vi "SelectPatternDialog.vi"(0 "GraphIn":refnum<class "Graph.lvclass">, 1 "SelectedNodes":refnum<class "AbstractNode.lvclass">[](array[class]), 5 "error in":errorcluster) -> (14 "GraphOut":refnum<class "Graph.lvclass">, 15 "Cancelled":bool, 16 "NodesOut":T3[](array[typedef]), 17 "LinksOut":T1[](array[typedef]), 18 "NodeIndexies":i32[](array[numeric]), 19 "error out":errorcluster)   [LabVIEW 2012]
uses:
  <resource>/Framework/Providers/Open_GDS/UML/Graph_class/Graph.lvclass
  <resource>/Framework/Providers/Open_GDS/UML/AbstractNode_class/AbstractNode.lvclass
  <resource>/Framework/Providers/Open_GDS/UML/DesignPattern/SubVIs/DesignPatterns_Node.ctl
  <resource>/Framework/Providers/Open_GDS/UML/DesignPattern/SubVIs/DesignPatterns_NodeType.ctl
  <resource>/Framework/Providers/Open_GDS/UML/DesignPattern/SubVIs/DesignPatterns_Link.ctl
  <resource>/Framework/Providers/Open_GDS/UML/DesignPattern/SubVIs/DesignPatterns_LinkType.ctl
  <resource>/Framework/Providers/Open_GDS/UML/Graphics_class/Graphics.lvclass
  <resource>/Framework/Providers/Open_GDS/UML/Grid_class/Grid.lvclass
  <resource>/Framework/Providers/Open_GDS/UML/ClassDiagramGraph_class/ClassDiagramGraph.lvclass
  <resource>/Framework/Providers/Open_GDS/UML/DesignPattern/SubVIs/DesignPatterns_Pattern.ctl
  <resource>/Framework/Providers/Open_GDS/UML/ClassNode_class/ClassNode.lvclass
  <resource>/Framework/Providers/Open_GDS/UML/Graphics_class/LvFontType.ctl
  <resource>/Framework/Providers/Open_GDS/UML/Graphics_class/FontType.ctl
  <resource>/Framework/Providers/Open_GDS/UML/DesignPattern/SubVIs/DesignPatterns_ClassNodeData.ctl
  <resource>/Framework/Providers/Open_GDS/UML/DesignPattern/SubVIs/DesignPatterns_Attribute.ctl
  <resource>/Framework/Providers/Open_GDS/UML/DesignPattern/SubVIs/DesignPatterns_Method.ctl
  <vilib>/Platform/browser.llb/Open URL in Default Browser (string).vi
panel:
  in  "OpenPatternFile":bool
  in  "Refresh":bool
  in  "Ring 10":u16(ring) items=["<Select>", "Handler", "ConcreteHandler1", "ConcreteHandler2", "Client"]
  in  "Ring 9":u16(ring) items=["<Select>", "Handler", "ConcreteHandler1", "ConcreteHandler2", "Client"]
  in  "Ring 8":u16(ring) items=["<Select>", "Handler", "ConcreteHandler1", "ConcreteHandler2", "Client"]
  in  "Ring 7":u16(ring) items=["<Select>", "Handler", "ConcreteHandler1", "ConcreteHandler2", "Client"]
  in  "Help":bool
  in  "Cancel":bool
  in  "OK":bool
  out "Nodes":cluster{"Name":string, "Desc":string}[](array[cluster])
  out "Pattern description":string
  out "NewVal":string
  in  "Design Patterns":string(tree)
  in  "InterfaceNames":string[](array[string])
  in  "PackageNames":string[](array[string])
  out "ClassNames":string[](array[string])
  in  "Ring 6":u16(ring) items=["<Select>", "Handler", "ConcreteHandler1", "ConcreteHandler2", "Client"]
  in  "Ring 5":u16(ring) items=["<Select>", "Handler", "ConcreteHandler1", "ConcreteHandler2", "Client"]
  in  "Ring 4":u16(ring) items=["<Select>", "Handler", "ConcreteHandler1", "ConcreteHandler2", "Client"]
  in  "Ring 3":u16(ring) items=["<Select>", "Handler", "ConcreteHandler1", "ConcreteHandler2", "Client"]
  in  "Ring 2":u16(ring) items=["<Select>", "Handler", "ConcreteHandler1", "ConcreteHandler2", "Client"]
  in  "Ring 1":u16(ring) items=["<Select>", "Handler", "ConcreteHandler1", "ConcreteHandler2", "Client"]
  out "Picture":picture
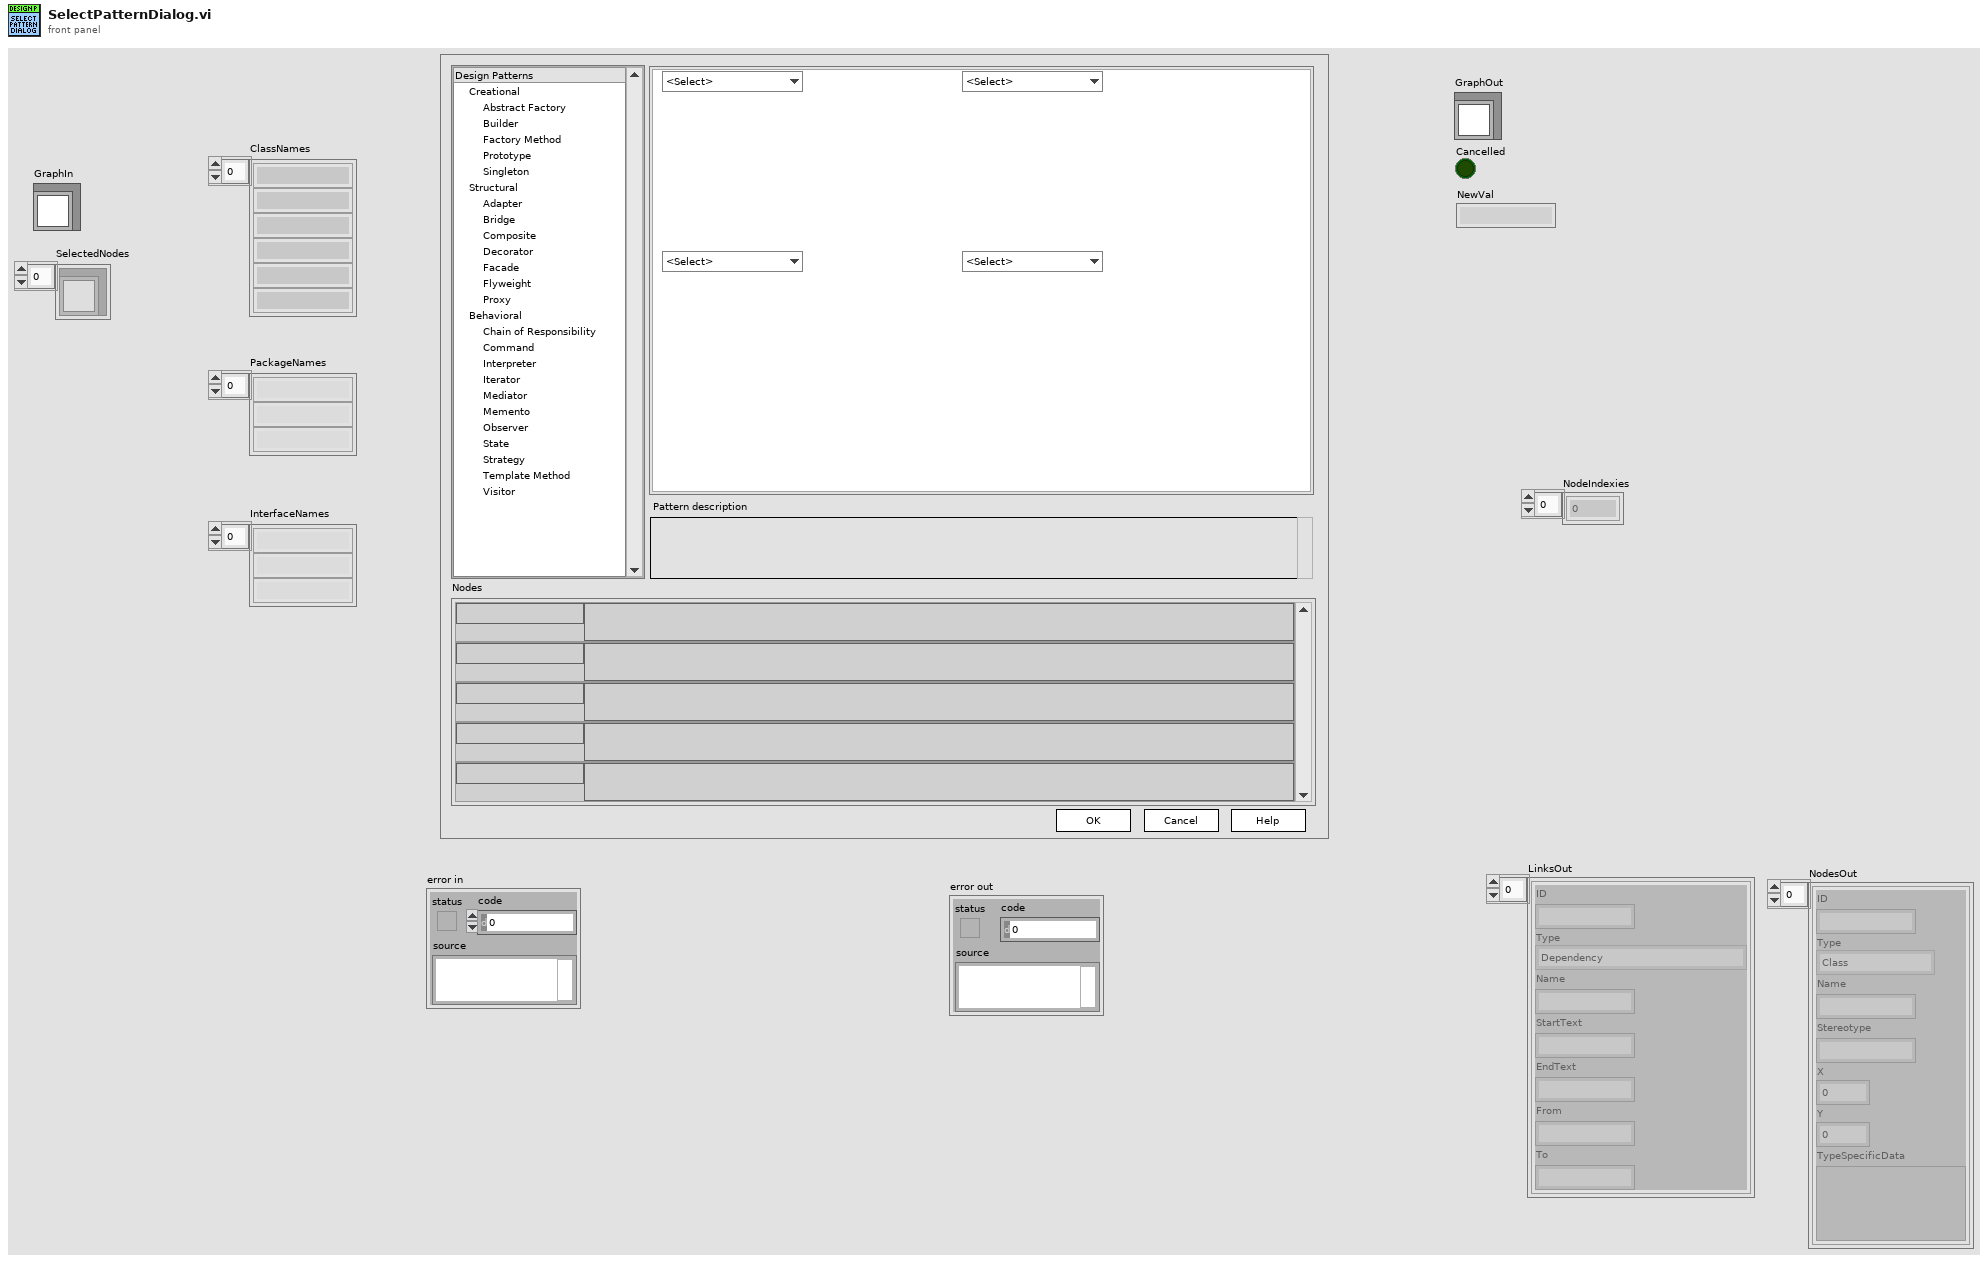
[diagram p1: front panel]
types:
  T1 = typedef "DesignPatterns_Link.ctl" = cluster{"ID":string, "Type":T2, "Name":string, "StartText":string, "EndText":string, "From":string, "To":string}
  T2 = typedef "DesignPatterns_LinkType.ctl" = enum16{"Dependency", "Inheritance", "Interface", "Association", "Aggregation", "CompositeAggregation"}
  T3 = typedef "DesignPatterns_Node.ctl" = cluster{"ID":string, "Type":T4, "Name":string, "Stereotype":string, "X":i32, "Y":i32, "TypeSpecificData":variant}
  T4 = typedef "DesignPatterns_NodeType.ctl" = enum16{"Class", "Interface", "Note", "Package"}
  T5 = typedef "DesignPatterns_Pattern.ctl" = cluster{"Version":string, "ID":string, "Name":string, "Category":string, "Help":string, "Desc":string}
  T6 = cluster{"Cancelled":bool, "Event":refnum<event-registration>, "CtrlRefs":refnum<vi>[], "PIDs":string[], "Graphics":refnum<class "Graphics.lvclass">, "Grid":refnum<class "Grid.lvclass">, "Diagram":refnum<class "ClassDiagramGraph.lvclass">, "ClassNodes":T3[], "ClassSelected":bool[], "NodeIndexies":i32[], "Patterns":cluster{"PatternFile":path, "Pattern":T5, "Nodes":T3[], "Links":T1[], "stripped path":path, "HelpExist":bool}[]}
  T7 = typedef "Graphics.lvclass/FontType.ctl" = cluster{"Font Name:":string, "Size":i16, "Strikeout?":bool, "Italic?":bool, "Underline?":bool, "Outline?":bool, "Shadow?":bool, "Bold?":bool}
  T8 = typedef "Graphics.lvclass/LvFontType.ctl" = enum16{"User-specified Font", "Application Font", "System Font", "Dialog Font"}
  T9 = cluster{path, "Pattern":T5, "Nodes":T3[], "Links":T1[], "stripped path":path, "file or folder exists?":bool}[]
  T10 = typedef "DesignPatterns_ClassNodeData.ctl" = cluster{"Description":string, "Attributes":T11[], "Methods":T12[]}
  T11 = typedef "DesignPatterns_Attribute.ctl" = cluster{"ID":string, "Name":string}
  T12 = typedef "DesignPatterns_Method.ctl" = cluster{"ID":string, "Name":string}
  T13 = typedef "Rectangle Rectangle2D.ctl" = cluster{"x":dbl, "y":dbl, "width":dbl, "height":dbl}
  T14 = cluster{path, "Pattern":T5, "Nodes":T3[], "Links":T1[], "stripped path":path, "file or folder exists?":bool}
  T15 = cluster{"PatternFile":path, "Pattern":T5, "Nodes":T3[], "Links":T1[], "stripped path":path, "HelpExist":bool}[]
  T16 = cluster{"PatternFile":path, "Pattern":T5, "Nodes":T3[], "Links":T1[], "stripped path":path, "HelpExist":bool}
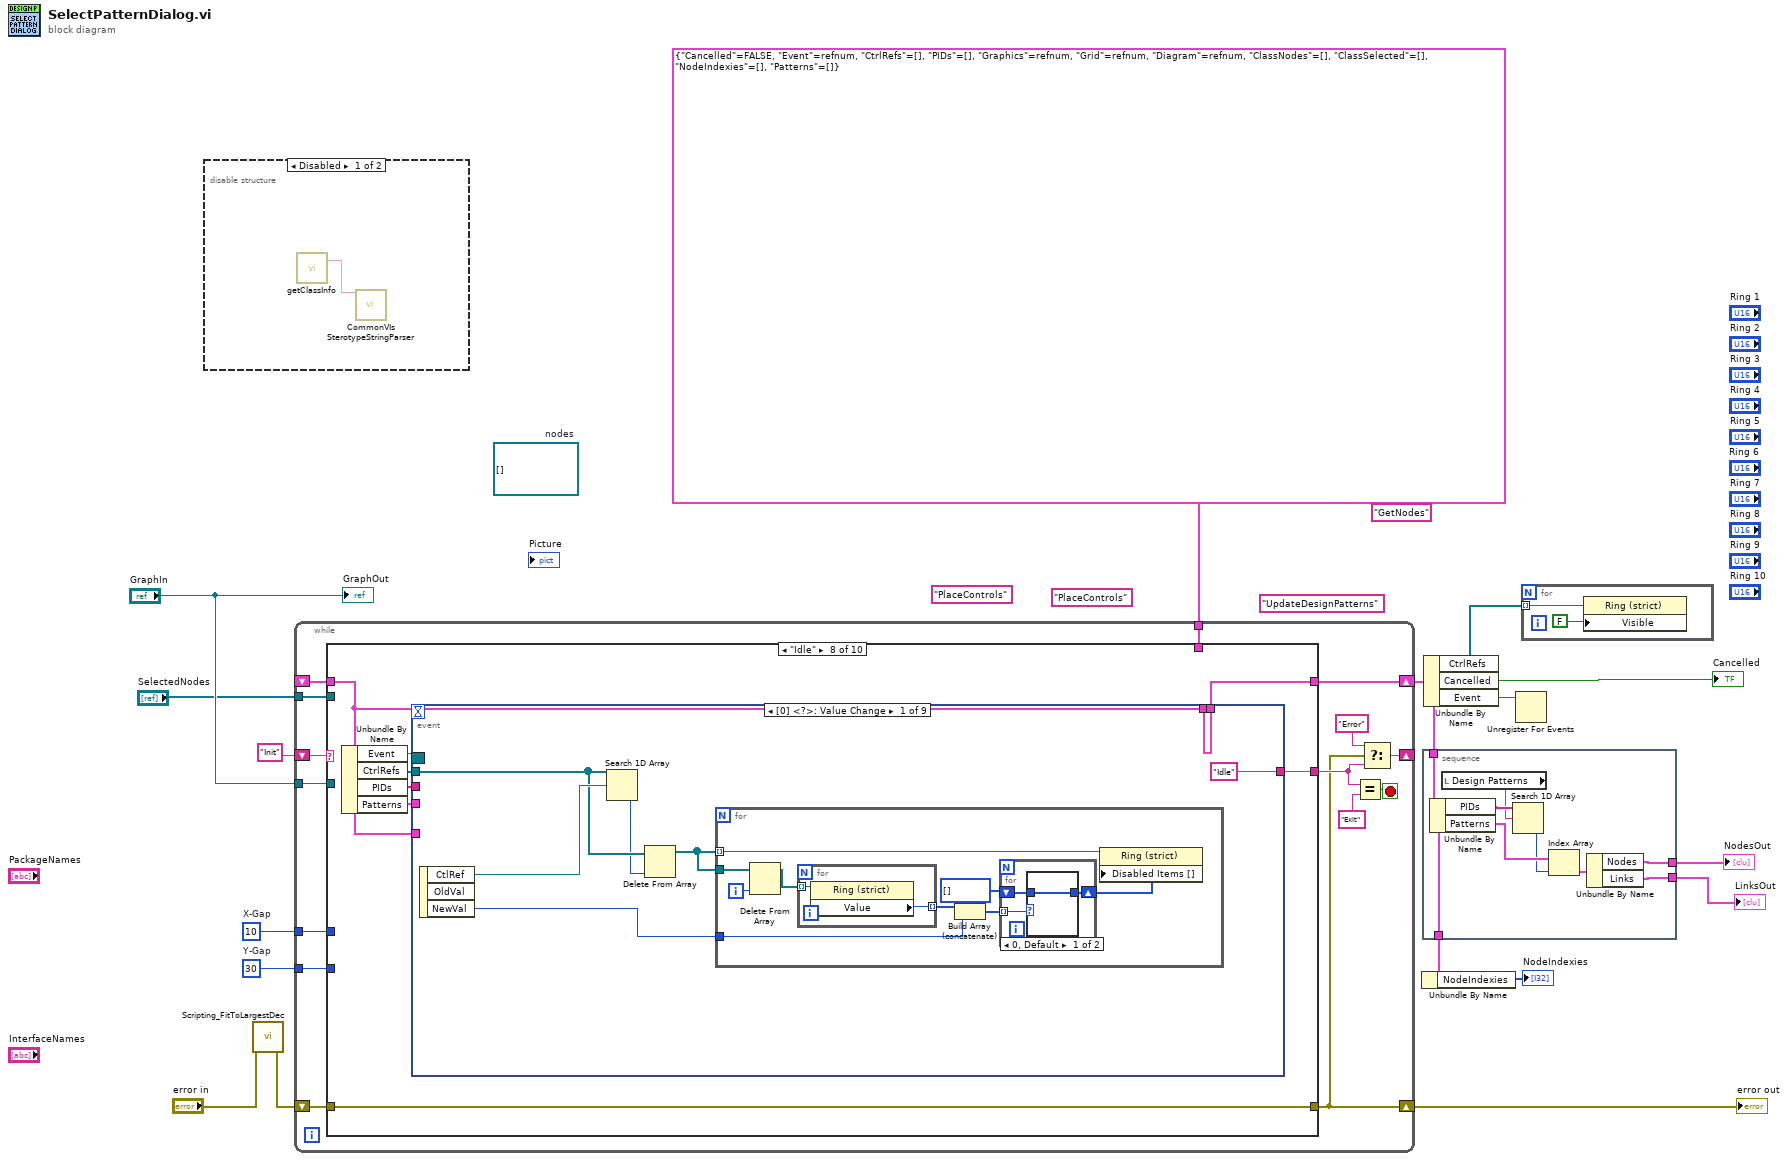
[diagram p0: block diagram]
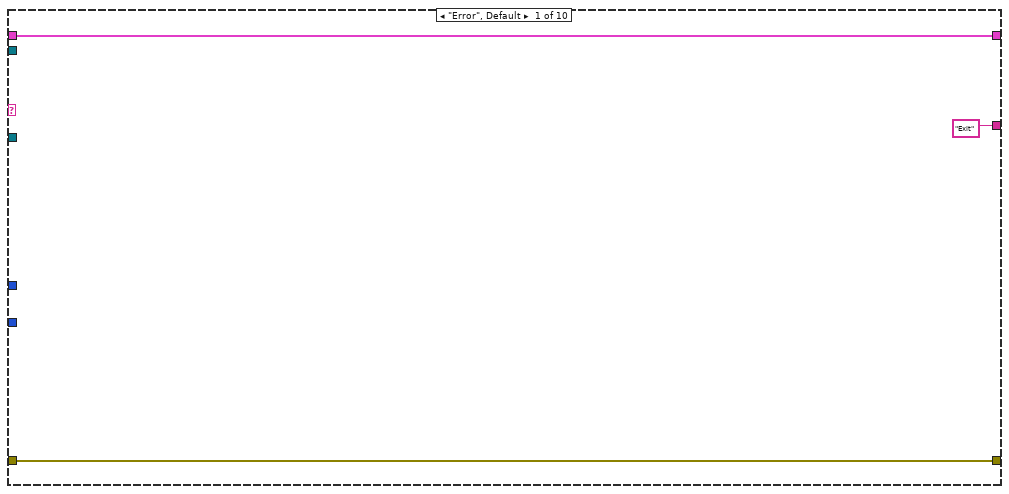
[diagram p3: hidden frame]
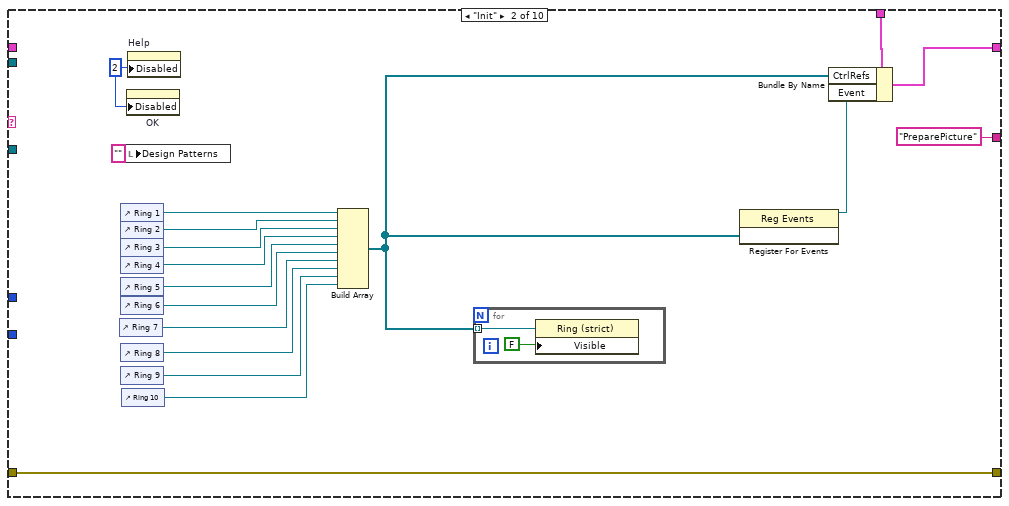
[diagram p4: hidden frame]
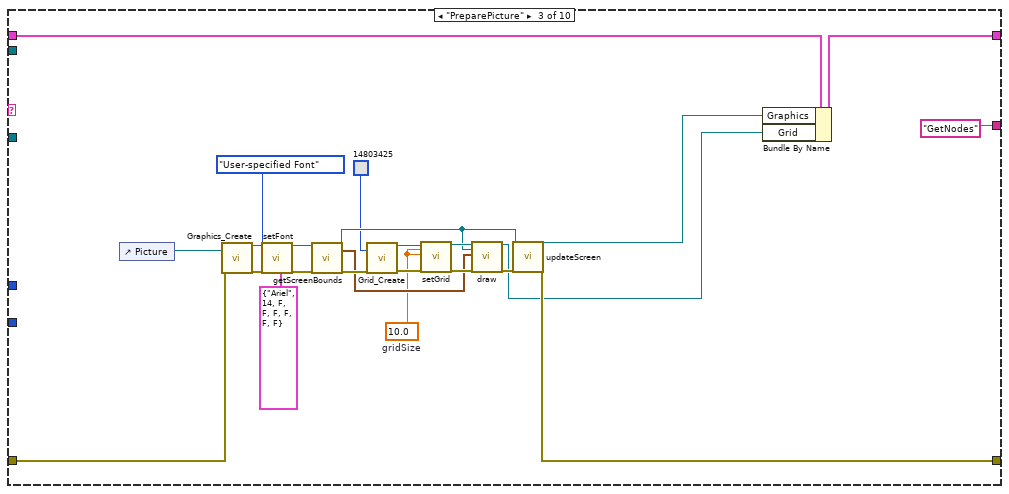
[diagram p5: hidden frame]
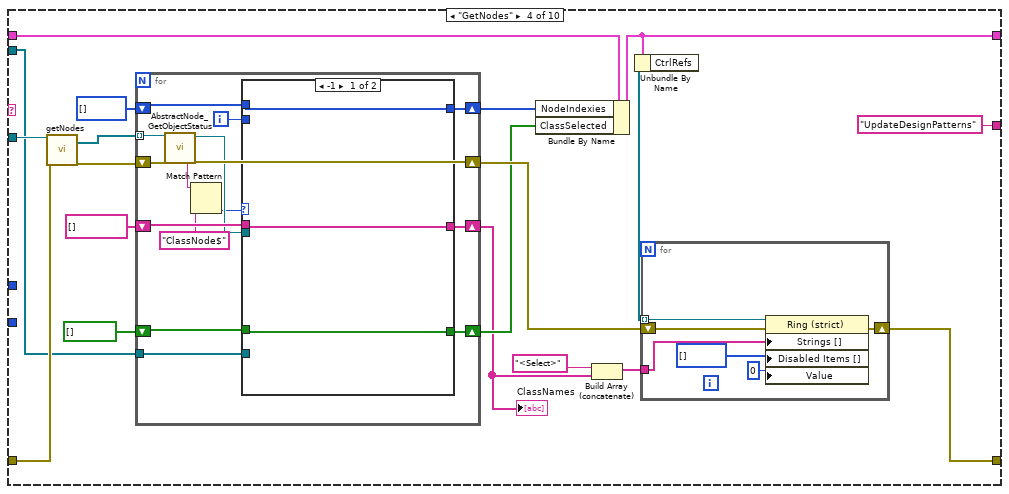
[diagram p6: hidden frame]
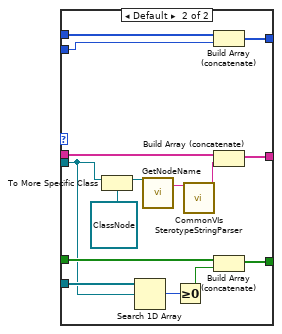
[diagram p7: hidden frame]
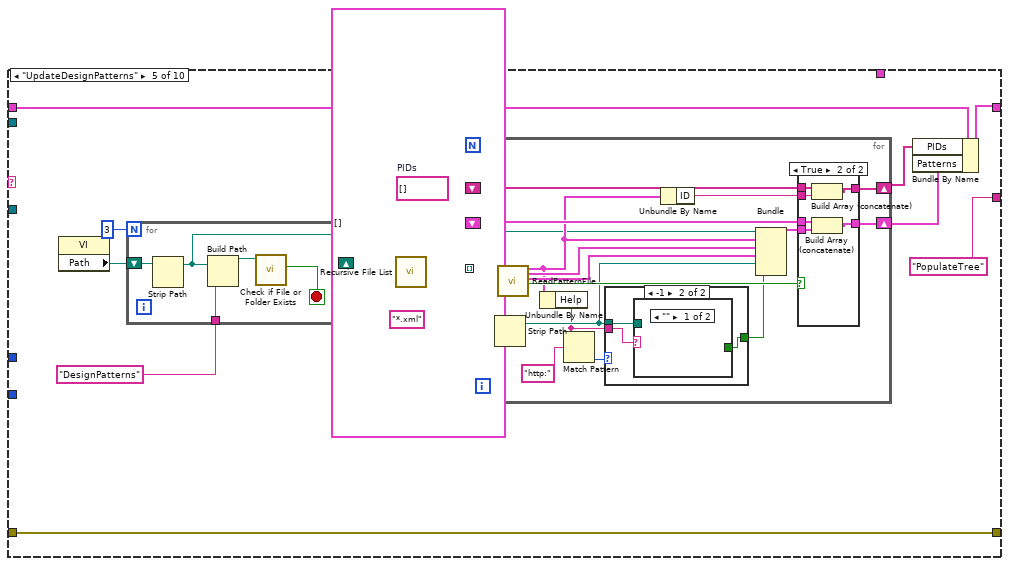
[diagram p8: hidden frame]
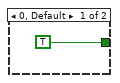
[diagram p9: hidden frame]
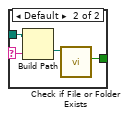
[diagram p10: hidden frame]
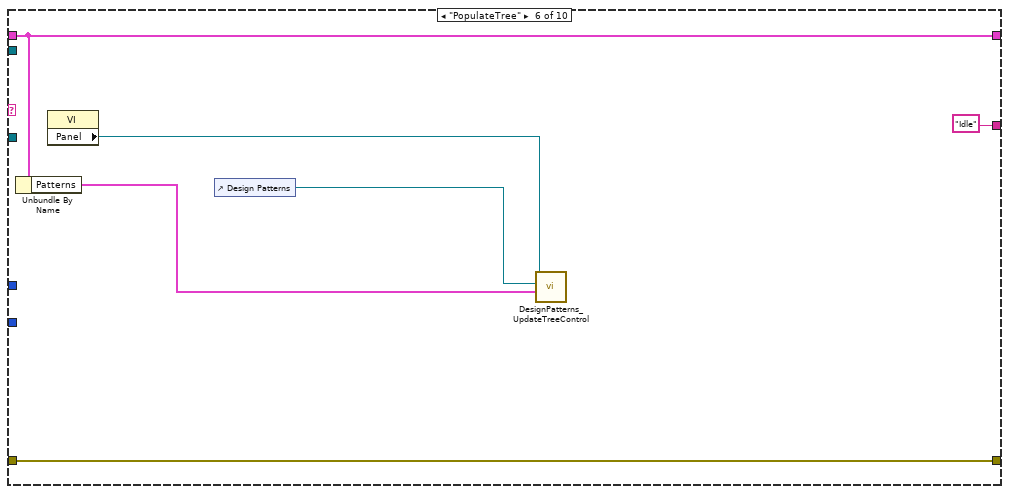
[diagram p12: hidden frame]
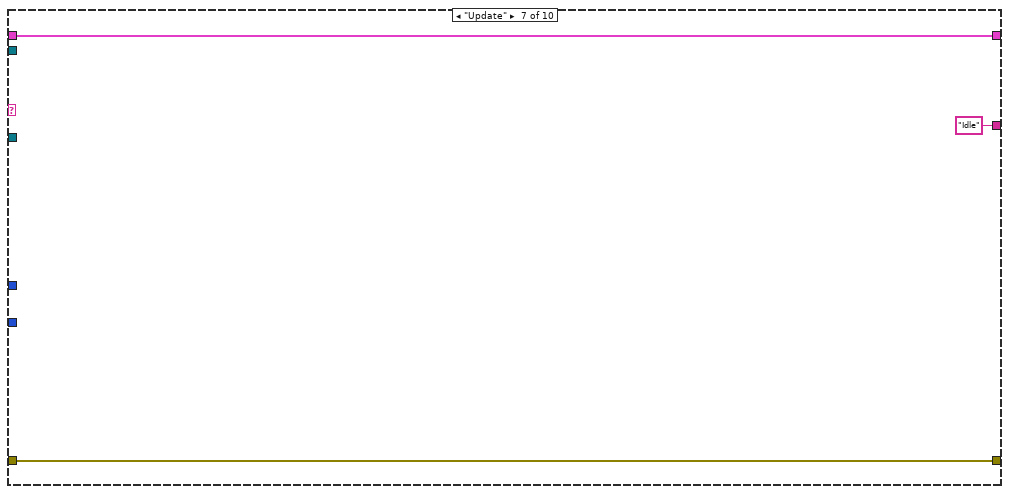
[diagram p13: hidden frame]
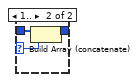
[diagram p14: hidden frame]
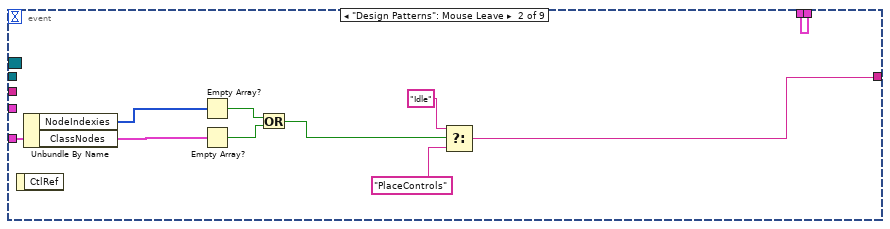
[diagram p15: hidden frame]
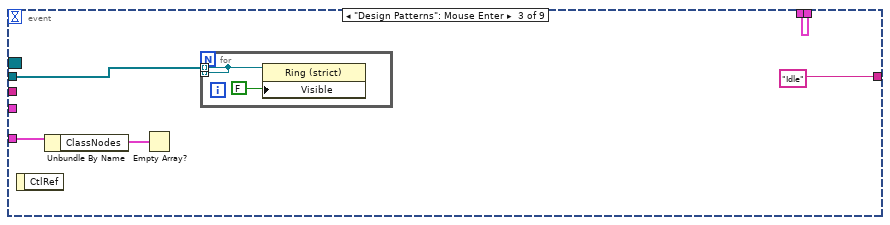
[diagram p16: hidden frame]
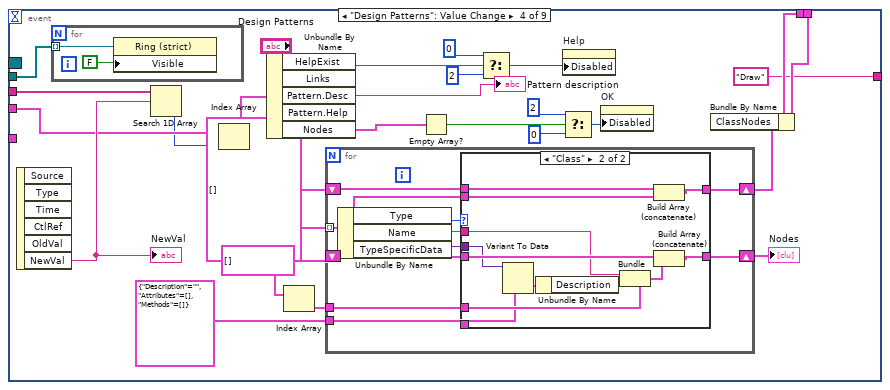
[diagram p17: hidden frame]
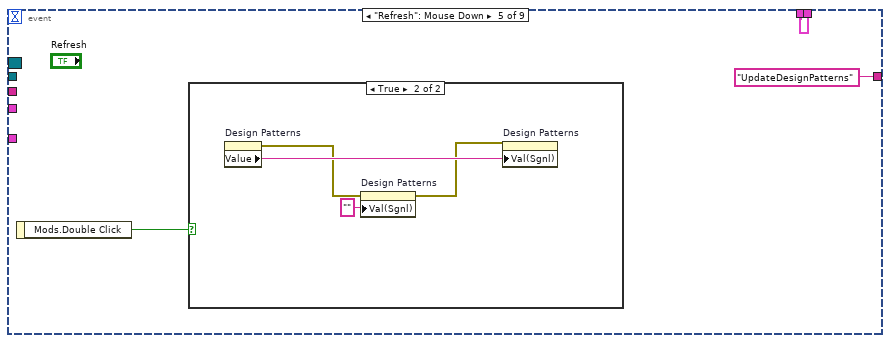
[diagram p19: hidden frame]
diagram:
  (unwired) "PlaceControls"
  w8 = 30  # Y-Gap
  w9 = 10  # X-Gap
  (unwired) refnum<class "ClassNode.lvclass">[] []  # nodes
  (unwired) "GetNodes"
  (unwired) "UpdateDesignPatterns"
  (unwired) "PlaceControls"
  n1 = disable-structure shown="Disabled" {
    frame Disabled {
      n2 = call-dynamic "getClassInfo.vi"() -> ("className"=w18:string, "ClassPath"=w19:path)  [unwired: 10 in, 8 out]
      n3 = call <resource>:"CommonVIs SterotypeStringParser.vi"("SterotypeStringIn"=w18) -> ()  [unwired: 19 out]
    }
    frame Enabled {
    }
  }
  n4 = call <resource>:"Scripting_FitToLargestDec.vi"("error in (no error)"="error in") -> ("error out"=w10:errorcluster)  [unwired: 5 in, 1 out]
  n5 = while {
    shift-right: [w27] -> w16
    shift-left: w10 -> [w34]
    shift-right: [w32] -> _
    shift-left: "Init" -> [w33]
    shift-right: [w26] -> w6
    shift-left: _ -> [w25]
    tunnel: T6 {"Cancelled"=FALSE, "Event"=refnum, "CtrlRefs"=[], "PIDs"=[], "Graphics"=refnum, "Grid"=refnum, "Diagram"=refnum, "ClassNodes"=[], "ClassSelected"=[], "NodeIndexies"=[], "Patterns"=[]} -> [w24]
    tunnel: "GraphIn" -> [w23]
    tunnel: w9 -> [w22]
    tunnel: w8 -> [w21]
    tunnel: "SelectedNodes" -> [w20]
    stop <- w31 stop-if-true
    n6 = case shown="\"Idle\"" w33 {
      tunnel: w34 -> [w37 w54 w65 w92 w143 w193 w197 w205 w373 w413]
      tunnel: [w37 w54 w64 w91 w143 w193 w197 w205 w375 w409] -> w27
      tunnel: ["Exit" "PreparePicture" "GetNodes" "UpdateDesignPatterns" "PopulateTree" "Idle" "Idle" w206 "Idle" "Idle"] -> w28
      tunnel: [w35 w53 w58 w86 w145 w195 w198 w207 w395 w407] -> w26
      tunnel: w25 -> [w35 _ w59 w87 w147 w195 w198 w200 w395 w407]
      tunnel: w24 -> [_ w45 _ _ _ _ _ _ _ _]
      tunnel: w23 -> [_ _ _ w94 _ _ _ _ _ _]
      tunnel: w22 -> [_ _ _ _ _ _ _ _ w368 w420]
      tunnel: w21 -> [_ _ _ _ _ _ _ _ w367 w419]
      tunnel: w20 -> [_ _ _ w89 _ _ _ _ _ w412]
      frame "Error", Default {
      }
      frame "Init" {
        w44 = u8 2 ("Disabled")
        n7 = control-ref of="Ring 7"() -> (w41:refnum<vi>)
        n8 = control-ref of="Ring 1"() -> (w47:refnum<vi>)
        n9 = control-ref of="Ring 2"() -> (w48:refnum<vi>)
        n10 = control-ref of="Ring 3"() -> (w49:refnum<vi>)
        n11 = control-ref of="Ring 4"() -> (w50:refnum<vi>)
        n12 = control-ref of="Ring 5"() -> (w51:refnum<vi>)
        n13 = control-ref of="Ring 6"() -> (w52:refnum<vi>)
        n14 = control-ref of="Ring 8"() -> (w40:refnum<vi>)
        n15 = control-ref of="Ring 9"() -> (w39:refnum<vi>)
        n16 = control-ref of="Ring 10"() -> (w38:refnum<vi>)
        n17 = local write "Design Patterns"("" ("Design Patterns")) -> ()
        n18 = property on="OK" class="Bool"("Disabled"=w44) -> ()  [unwired: 2 in, 2 out]
        n19 = property on="Help" class="Bool"("Disabled"=w44) -> ()  [unwired: 2 in, 2 out]
        n20 = Build Array(w47, w48, w49, w50, w51, w52, w41, w40, w39, w38) -> (w42:refnum<vi>[])
        n21 = for {
          tunnel: w42 -> [w57] mode=indexing
          n22 = property class="Ring (strict)"(reference=w57, "Visible"=FALSE) -> ()  [unwired: 1 in, 2 out]
        }
        n23 = register-events(w42) -> (reference out=w46:refnum<event-registration>)  [unwired: 2 in, 1 out]
        n24 = Bundle By Name(cluster=w45, "CtrlRefs"=w42, "Event"=w46) -> (w53:T6)
      }
      frame "PreparePicture" {
        w66 = 10.0  # gridSize
        n25 = control-ref of="Picture"() -> (w62:refnum<vi>)
        n26 = call <resource>:"Graphics_Create.vi"("screenRef"=w62, "error in (no error)"=w65) -> ("reference out"=w75:refnum<class "Graphics.lvclass">, "error out"=w74:errorcluster)  [unwired: 2 in, 14 out]
        n27 = call <resource>:"setFont.vi"("reference"=w75, "fontType"=LvFontType."User-specified Font", "font"=T7 {"Font Name:"="Ariel", "Size"=14, "Strikeout?"=FALSE, "Italic?"=FALSE, "Underline?"=FALSE, "Outline?"=FALSE, "Shadow?"=FALSE, "Bold?"=FALSE}, "error in (no error)"=w74) -> ("reference out"=w73:refnum<class "Graphics.lvclass">, "error out"=w72:errorcluster)  [unwired: 14 out]
        n28 = call <resource>:"getScreenBounds.vi"("reference"=w73, "error in (no error)"=w72) -> ("reference out"=w76:refnum<class "Graphics.lvclass">, "bounds"=w69:T13, "error out"=w81:errorcluster)  [unwired: 15 out]
        n29 = call <resource>:"Grid_Create.vi"("gridColor"=u32 14803425, "error in (no error)"=w81) -> ("reference out"=w78:refnum<class "Grid.lvclass">, "error out"=w79:errorcluster)  [unwired: 2 in, 14 out]
        n30 = call <resource>:"setGrid.vi"("reference"=w78, "gridX"=w66, "gridY"=w66, "error in (no error)"=w79) -> ("reference out"=w77:refnum<class "Grid.lvclass">, "error out"=w80:errorcluster)  [unwired: 14 out]
        n31 = call-dynamic "draw.vi"("reference"=w77, "graphics"=w76, "bounds"=w69, "error in (no error)"=w80) -> ("reference out"=w60:refnum<class "Grid.lvclass">, "error out"=w68:errorcluster)  [unwired: 14 in]
        n32 = call <resource>:"updateScreen.vi"("reference"=w76, "error in (no error)"=w68) -> ("reference out"=w61:refnum<class "Graphics.lvclass">, "error out"=w64:errorcluster)  [unwired: 16 out]
        n33 = Bundle By Name(cluster=w59, "Graphics"=w61, "Grid"=w60) -> (w58:T6)
      }
      frame "GetNodes" {
        n34 = call-dynamic "getNodes.vi"("reference"=w94, "error in (no error)"=w92) -> ("nodes"=w93:refnum<class "AbstractNode.lvclass">[], "error out"=w96:errorcluster)  [unwired: 15 in, 1 out]
        n35 = for {
          shift-right: [w113] -> w90
          shift-left: w96 -> [w115]
          tunnel: w93 -> [w114] mode=indexing
          shift-right: [w110] -> w82
          shift-left: string[] [] ("nodes") -> [w112]
          shift-right: [w106] -> w85
          shift-left: bool[] [] -> [w105]
          tunnel: w89 -> [w104]
          shift-right: [w103] -> w83
          shift-left: i32[] [] -> [w102]
          i -> [w101]
          n36 = call <resource>:"AbstractNode_GetObjectStatus.vi"("reference in"=w114, "error in (no error)"=w115) -> ("Class name"=w109:string, "reference out"=w111:refnum<class "AbstractNode.lvclass">, "error out"=w113:errorcluster)  [unwired: 15 out]
          n37 = Match Pattern(string=w109, regular expression="ClassNode$") -> (offset past match=w107:i32)  [unwired: 4 out]
          n38 = case shown="-1" w107 {
            tunnel: w112 -> [w118 w133]
            tunnel: w111 -> [_ w124]
            tunnel: [w118 w132] -> w110
            tunnel: [w117 w127] -> w106
            tunnel: w105 -> [w117 w126]
            tunnel: w104 -> [_ w125]
            tunnel: [w116 w121] -> w103
            tunnel: w102 -> [w116 w120]
            tunnel: w101 -> [_ w119]
            frame -1 {
            }
            frame Default {
              n39 = To More Specific Class(target class=refnum<class "ClassNode.lvclass"> refnum ("reference"), reference=w124) -> (specific class reference=w130:refnum<class "ClassNode.lvclass">)  [unwired: 1 in, 1 out]
              n40 = Search 1D Array(1D array=w125, element=w124) -> (index of element=w123:i32)  [unwired: 1 in]
              n41 = call-dynamic "GetNodeName.vi"("reference in"=w130) -> ("String"=w129:string)  [unwired: 16 in, 2 out]
              n42 = Greater Or Equal To 0?(x=w123) -> (x >= 0?=w122:bool)
              n43 = call <resource>:"CommonVIs SterotypeStringParser.vi"("SterotypeStringIn"=w129) -> ("Name"=w128:string)  [unwired: 18 out]
              n44 = Build Array (concatenate)(w120, w119) -> (w121:i32[])
              n45 = Build Array (concatenate)(w133, w128) -> (w132:string[])
              n46 = Build Array (concatenate)(w126, w122) -> (w127:bool[])
            }
          }
        }
        "ClassNames" <- w82
        n47 = Bundle By Name(cluster=w87, "NodeIndexies"=w83, "ClassSelected"=w85) -> (w86:T6)
        n48 = Build Array (concatenate)("<Select>", w82) -> (w99:string[])
        n49 = Unbundle By Name(w86) -> ("CtrlRefs"=w98:refnum<vi>[])
        n50 = for {
          tunnel: w98 -> [w139] mode=indexing
          tunnel: w99 -> [w138]
          shift-right: [w134] -> w91
          shift-left: w90 -> [w135]
          n51 = property class="Ring (strict)"(reference=w139, error in=w135, "Strings []"=w138, "Disabled Items []"=i32[] [], "Value"=u16 0) -> (error out=w134:errorcluster)  [unwired: 1 out]
        }
      }
      frame "UpdateDesignPatterns" {
        w142 = string[] []  # PIDs
        n52 = property class="VI"() -> ("Path"=w151:path)  [unwired: 2 in, 2 out]
        n53 = for {
          N: 3 -> [_]
          tunnel: "DesignPatterns" ("name or relative path") -> [w190]
          shift-right: [w186] -> w150
          shift-left: w151 -> [w187]
          stop <- w188 stop-if-true
          n54 = Strip Path(path=w187) -> (stripped path=w186:path)  [unwired: 1 out]
          n55 = Build Path(base path=w186, name or relative path=w190) -> (appended path=w189:path)
          n56 = call <vilib>:"Check if File or Folder Exists.vi"("path"=w189) -> ("file or folder exists?"=w188:bool)  [unwired: 1 in, 9 out]
        }
        n57 = call <vilib>:"Recursive File List.vi"("pattern"="*.xml", "Folder Path"=w150) -> ("All Files in Dir"=w148:path[])  [unwired: 2 in, 7 out]
        n58 = for {
          tunnel: w148 -> [w154] mode=indexing
          shift-right: [w165] -> w146
          shift-left: T9 [] -> [w167]
          shift-right: [w162] -> w141
          shift-left: w142 -> [w161]
          n59 = Strip Path(path=w154) -> (stripped path=w156:path)  [unwired: 1 out]
          n60 = call <resource>:"ReadPatternFile.vi"("PatternsXMLFileIn"=w154) -> ("Pattern"=w160:T5, "Nodes"=w169:T3[], "Links"=w168:T1[], "Valid"=w164:bool)  [unwired: 2 in, 13 out]
          n61 = Unbundle By Name(w160) -> ("Help"=w155:string)
          n62 = Match Pattern(string=w155, regular expression="http:") -> (offset past match=w158:i32)  [unwired: 4 out]
          n63 = case shown="-1" w158 {
            tunnel: [TRUE w171] -> w157
            tunnel: w156 -> [_ w173]
            tunnel: w155 -> [_ w172]
            frame 0, Default {
            }
            frame -1 {
              n64 = case shown="\"\"" w172 {
                selector: w172 -> [_ w175]
                tunnel: w173 -> [_ w176]
                tunnel: [_ w174] -> w171
                frame "" {
                }
                frame Default {
                  n65 = Build Path(base path=w176, name or relative path=w175) -> (appended path=w177:path)
                  n66 = call <vilib>:"Check if File or Folder Exists.vi"("path"=w177) -> ("file or folder exists?"=w174:bool)  [unwired: 1 in, 9 out]
                }
              }
            }
          }
          n67 = Unbundle By Name(w160) -> ("ID"=w163:string)
          n68 = Bundle(w154, "Pattern"=w160, "Nodes"=w169, "Links"=w168, "stripped path"=w156, "file or folder exists?"=w157) -> (w166:T14)  [unwired: 1 out]
          n69 = case shown="True" w164 {
            tunnel: w167 -> [w179 w185]
            tunnel: w166 -> [_ w184]
            tunnel: [w179 w183] -> w165
            tunnel: w163 -> [_ w182]
            tunnel: [w178 w181] -> w162
            tunnel: w161 -> [w178 w180]
            frame False {
            }
            frame True {
              n70 = Build Array (concatenate)(w180, w182) -> (w181:string[])
              n71 = Build Array (concatenate)(w185, w184) -> (w183:T9)
            }
          }
        }
        n72 = Bundle By Name(cluster=w147, "PIDs"=w141, "Patterns"=w146) -> (w145:T6)
      }
      frame "PopulateTree" {
        n73 = Unbundle By Name(w195) -> ("Patterns"=w192:T15)
        n74 = property class="VI"() -> ("Panel"=w196:refnum<vi>)  [unwired: 2 in, 2 out]
        n75 = control-ref of="Design Patterns"() -> (w191:refnum<vi>)
        n76 = call <resource>:"DesignPatterns_UpdateTreeControl.vi"("Patterns"=w192, "Tree Refnum"=w191, "Panel"=w196) -> ()  [unwired: 9 out]
      }
      frame "Update" {
      }
      frame "Idle" {
        n77 = Unbundle By Name(w200) -> ("Event"=w204:refnum<event-registration>, "CtrlRefs"=w203:refnum<vi>[], "PIDs"=w202:string[], "Patterns"=w201:T15)
        n78 = event shown="[0] <?>: Value Change" {
          selector: w204 -> [_ _ _ _ _ _ _ _ _]
          dyn-events: _ -> [_ _ _ _ _ _ _ _ _]
          timeout: _ -> [_ _ _ _ _ _ _ _ _]
          tunnel: w200 -> [w209 w242 w245 w255 w302 w309 w324 w341 w351]
          tunnel: [w209 w242 w245 w254 w302 w309 w324 w340 w350] -> w207
          tunnel: ["Idle" w237 "Idle" ("t") "Draw" "UpdateDesignPatterns" "Idle" ("t") "Idle" "Exit" "Exit"] -> w206
          tunnel: w203 -> [w213 _ w243 w256 _ _ _ _ _]
          tunnel: w202 -> [_ _ _ w274 _ w311 w331 _ _]
          tunnel: w201 -> [_ _ _ w272 _ w310 w329 _ _]
          tunnel: w200 -> [_ w241 w246 _ _ _ _ _ w347]
          event Value Change {
            n79 = event-data() -> ("CtlRef"=w214:refnum<vi>, "NewVal"=w210:u16)  [unwired: 2 out]
            n80 = Search 1D Array(1D array=w213, element=w214) -> (index of element=w212:i32)  [unwired: 1 out]
            n81 = Delete From Array(array=w213, index=w212) -> (array with subset deleted=w211:refnum<vi>[])  [unwired: 1 in, 1 out]
            n82 = for {
              tunnel: w211 -> [w223] mode=indexing
              tunnel: w211 -> [w222]
              tunnel: w210 -> [w218]
              i -> [w221]
              n83 = Delete From Array(array=w222, index=w221) -> (array with subset deleted=w220:refnum<vi>[])  [unwired: 1 in, 1 out]
              n84 = for {
                tunnel: w220 -> [w232] mode=indexing
                tunnel: [w231] -> w219 mode=indexing
                n85 = property class="Ring (strict)"(reference=w232) -> ("Value"=w231:u16)  [unwired: 1 in, 2 out]
              }
              n86 = Build Array (concatenate)(w219, w218) -> (w217:u16[])
              n87 = for {
                tunnel: w217 -> [w226] mode=indexing
                shift-right: [w224] -> w215
                shift-left: u16[] [] -> [w225]
                n88 = case shown="0, Default" w226 {
                  selector: w226 -> [_ w228]
                  tunnel: w225 -> [w227 w230]
                  tunnel: [w227 w229] -> w224
                  frame 0, Default {
                  }
                  frame 1.. {
                    n89 = Build Array (concatenate)(w230, w228) -> (w229:u16[])
                  }
                }
              }
              n90 = property class="Ring (strict)"(reference=w223, "Disabled Items []"=w215) -> ()  [unwired: 1 in, 2 out]
            }
          }
          event "Design Patterns": Mouse Leave {
            n91 = event-data() -> ()  [unwired: 2 out]
            n92 = Unbundle By Name(w241) -> ("NodeIndexies"=w236:i32[], "ClassNodes"=w240:T3[])
            n93 = Empty Array?(array=w236) -> (empty?=w235:bool)
            n94 = Empty Array?(array=w240) -> (empty?=w234:bool)
            n95 = Or(x=w235, y=w234) -> (x .or. y?=w233:bool)
            n96 = Select(t="Idle", s=w233, f="PlaceControls") -> (s? t:f=w237:string)
          }
          event "Design Patterns": Mouse Enter {
            n97 = event-data() -> ()  [unwired: 2 out]
            n98 = Unbundle By Name(w246) -> ("ClassNodes"=w247:T3[])
            n99 = Empty Array?(array=w247) -> ()  [unwired: 1 out]
            n100 = for {
              tunnel: [w248] -> _ mode=indexing
              tunnel: w243 -> [w248] mode=indexing
              n101 = property class="Ring (strict)"(reference=w248, "Visible"=FALSE) -> ()  [unwired: 1 in, 2 out]
            }
          }
          event "Design Patterns": Value Change {
            w269 = cluster{"Name":string, "Desc":string}[] [] ("Nodes")
            n102 = event-data() -> ("NewVal"=w273:string)  [unwired: 6 out]
            "NewVal" <- w273
            n103 = for {
              tunnel: w256 -> [w276] mode=indexing
              n104 = property class="Ring (strict)"(reference=w276, "Visible"=FALSE) -> ()  [unwired: 1 in, 2 out]
            }
            n105 = Search 1D Array(1D array=w274, element=w273) -> (index of element=w271:i32)  [unwired: 1 out]
            n106 = Index Array(array=w272, index=w271) -> (element=w270:T16)
            n107 = Unbundle By Name(w270) -> ("HelpExist"=w265:bool, "Pattern.Desc"=→"Pattern description":string, "Nodes"=w259:T3[])  [unwired: 2 out]
            n108 = Index Array(array=w269) -> (element=w268:cluster{"Name":string, "Desc":string})  [unwired: 1 in]
            n109 = for {
              tunnel: w259 -> [w278] mode=indexing
              shift-right: [w283] -> w266
              shift-left: w269 -> [w284]
              tunnel: w268 -> [w285]
              tunnel: T10 {"Description"="", "Attributes"=[], "Methods"=[]} -> [w281]
              shift-right: [w277] -> w251
              shift-left: T3[] [] -> [w279]
              n110 = Unbundle By Name(w278) -> ("Type"=w286:T4, "Name"=w282:string, "TypeSpecificData"=w280:variant)
              n111 = case shown="\"Class\"" w286 {
                tunnel: w285 -> [_ w300]
                tunnel: w284 -> [w288 w299]
                tunnel: [w288 w297] -> w283
                tunnel: w282 -> [_ w296]
                tunnel: w281 -> [_ w295]
                tunnel: w280 -> [_ w294]
                tunnel: w279 -> [w287 w291]
                tunnel: w278 -> [_ w290]
                tunnel: [w287 w289] -> w277
                frame Default {
                }
                frame "Class" {
                  n112 = Variant To Data(type=w295, Variant=w294) -> (data=w293:T10)  [unwired: 1 in, 1 out]
                  n113 = Unbundle By Name(w293) -> ("Description"=w292:string)
                  n114 = Bundle(cluster=w300, "Name"=w296, "Desc"=w292) -> (w298:cluster{"Name":string, "Desc":string})
                  n115 = Build Array (concatenate)(w291, w290) -> (w289:T3[])
                  n116 = Build Array (concatenate)(w299, w298) -> (w297:cluster{"Name":string, "Desc":string}[])
                }
              }
            }
            "Nodes" <- w266
            n117 = Empty Array?(array=w259) -> (empty?=w257:bool)
            n118 = Select(t=u8 0 ("Disabled"), s=w265, f=u8 2 ("Disabled")) -> (s? t:f=w264:u8)
            n119 = property on="Help" class="Bool"("Disabled"=w264) -> ()  [unwired: 2 in, 2 out]
            n120 = Select(t=u8 2 ("Disabled"), s=w257, f=u8 0 ("Disabled")) -> (s? t:f=w258:u8)
            n121 = property on="OK" class="Bool"("Disabled"=w258) -> ()  [unwired: 2 in, 2 out]
            n122 = Bundle By Name(cluster=w255, "ClassNodes"=w251) -> (w254:T6)
          }
          event "Refresh": Mouse Down {
            n123 = event-data() -> ("Mods.Double Click"=w301:bool)  [unwired: 1 out]
            n124 = case shown="True" w301 {
              frame False {
              }
              frame True {
                n125 = property on="Design Patterns" class="Tree (strict)"() -> (error out=w306:errorcluster, "Value"=w307:string)  [unwired: 2 in, 1 out]
                n126 = property on="Design Patterns" class="Tree (strict)"(error in=w306, "Val(Sgnl)"="" ("Value (Signaling)")) -> (error out=w305:errorcluster)  [unwired: 1 in, 1 out]
                n127 = property on="Design Patterns" class="Tree (strict)"(error in=w305, "Val(Sgnl)"=w307) -> ()  [unwired: 1 in, 2 out]
              }
            }
          }
          event "OpenPatternFile": Mouse Down {
            n128 = event-data() -> ("Mods.Double Click"=w312:bool)  [unwired: 1 out]
            n129 = case shown="True" w312 {
              tunnel: w311 -> [_ w320]
              tunnel: w310 -> [_ w318]
              frame False {
              }
              frame True {
                n130 = local read "NewVal"() -> (w319:string)
                n131 = Search 1D Array(1D array=w320, element=w319) -> (index of element=w321:i32)  [unwired: 1 out]
                n132 = Index Array(array=w318, index=w321) -> (element=w317:T16)
                n133 = Unbundle By Name(w317) -> ("PatternFile"=w316:path)
                n134 = Format Into String(format string="notepad \"%s\"", w316) -> (resulting string=w314:string)  [unwired: 2 in, 1 out]
                n135 = call <vilib>:"System Exec.vi"("wait until completion? (T)"=FALSE, "command line"=w314) -> ()  [unwired: 6 in, 4 out]
              }
            }
          }
          event "Help": Value Change {
            n136 = event-data() -> ()  [unwired: 7 out]
            n137 = local read "Design Patterns"() -> (w330:string)
            n138 = Search 1D Array(1D array=w331, element=w330) -> (index of element=w333:i32)  [unwired: 1 out]
            n139 = Index Array(array=w329, index=w333) -> (element=w332:T16)
            n140 = Unbundle By Name(w332) -> ("stripped path"=w322:path, "Pattern.Help"=w326:string)
            n141 = Match Pattern(string=w326, regular expression="http:") -> (offset past match=w327:i32)  [unwired: 4 out]
            n142 = case shown="-1" w327 {
              tunnel: w326 -> [w334 w337]
              tunnel: [w334 w335] -> w325
              tunnel: w322 -> [_ w338]
              frame 0, Default {
              }
              frame -1 {
                n143 = Build Path(base path=w338, name or relative path=w337) -> (appended path=w336:path)
                n144 = Path To String(path=w336) -> (string=w335:string)
              }
            }
            n145 = call-poly <vilib>:"Open URL in Default Browser.vi"("URL"=w325) -> ()  [unwired: 1 in, 6 out]
          }
          event Panel Close? {
            w339 = TRUE ("Discard?")
            n146 = event-data() -> ()  [unwired: 2 out]
            n147 = Bundle By Name(cluster=w341, "Cancelled"=w339) -> (w340:T6)
            n148 = event-data("Discard?"=w339) -> ()  [unwired: 1 in, 1 out]
          }
          event "Cancel", "OK": Value Change {
            n149 = event-data() -> ()  [unwired: 4 out]
            n150 = Unbundle By Name(w347) -> ("CtrlRefs"=w346:refnum<vi>[], "ClassNodes"=w345:T3[], "NodeIndexies"=w344:i32[])
            n151 = case shown="True" "OK" {
              tunnel: w346 -> [_ w356]
              tunnel: w345 -> [_ w355]
              tunnel: w344 -> [_ w354]
              tunnel: [_ w353] -> w343
              frame False {
              }
              frame True {
                n152 = for {
                  tunnel: w356 -> [w360] mode=indexing
                  tunnel: w355 -> [_] mode=indexing
                  tunnel: w354 -> [w359]
                  tunnel: [w357] -> w353 mode=indexing
                  n153 = property class="Ring (strict)"(reference=w360) -> ("Value"=w358:u16)  [unwired: 1 in, 2 out]
                  n154 = case shown="1.." w358 {
                    selector: w358 -> [_ w363]
                    tunnel: w359 -> [_ w365]
                    tunnel: [-1 w362] -> w357
                    frame 0, Default {
                    }
                    frame 1.. {
                      n155 = Decrement(x=w363) -> (x-1=w364:u16)
                      n156 = Index Array(array=w365, index=w364) -> (element=w362:i32)
                    }
                  }
                }
              }
            }
            n157 = Bundle By Name(cluster=w351, "Cancelled"="Cancel", "NodeIndexies"=w343) -> (w350:T6)
          }
        }
      }
      frame "Draw" {
        w370 = 1000
        w384 = 0.0 ("x")
        n158 = Unbundle By Name(w395) -> ("Graphics"=w379:refnum<class "Graphics.lvclass">, "Grid"=w381:refnum<class "Grid.lvclass">)
        n159 = Unbundle By Name(w395) -> ("PIDs"=w399:string[], "Patterns"=w398:T15)  [unwired: 1 out]
        n160 = local read "Design Patterns"() -> (w400:string)
        n161 = call <resource>:"ClassDiagramGraph_Create.vi"("error in (no error)"=w373) -> ("reference out"=w371:refnum<class "ClassDiagramGraph.lvclass">, "error out"=w372:errorcluster)  [unwired: 2 in, 15 out]
        n162 = Search 1D Array(1D array=w399, element=w400) -> (index of element=w402:i32)  [unwired: 1 out]
        n163 = Index Array(array=w398, index=w402) -> (element=w401:T16)
        n164 = Unbundle By Name(w401) -> ("Nodes"=w397:T3[], "Links"=w396:T1[])
        n165 = call <resource>:"DesignPatterns_DrawNodesAndLinks.vi"("GraphIn"=w371, "Graphics"=w379, "Grid"=w381, "Nodes"=w397, "Links"=w396, "error in (no error)"=w372, "Y-Offset"=w367, "X-Offset"=w368) -> ("GraphOut"=w394:refnum<class "ClassDiagramGraph.lvclass">, "error out"=w380:errorcluster)  [unwired: 9 in, 1 out]
        n166 = call-dynamic "layout.vi"("reference"=w394, "error in (no error)"=w380) -> ("reference out"=w385:refnum<class "ClassDiagramGraph.lvclass">, "error out"=w386:errorcluster)  [unwired: 16 in]
        n167 = call <resource>:"resetPicture.vi"("reference"=w379, "error in (no error)"=w386) -> ("reference out"=w392:refnum<class "Graphics.lvclass">, "error out"=w391:errorcluster)  [unwired: 16 out]
        n168 = call <resource>:"getScreenBounds.vi"("reference"=w392, "error in (no error)"=w391) -> ("reference out"=w369:refnum<class "Graphics.lvclass">, "bounds"=w389:T13, "ZoomChanged"=w388:bool, "error out"=w390:errorcluster)  [unwired: 14 out]
        n169 = Bundle(cluster=w389, "x"=w384, "y"=w384, "width"=w370, "height"=w370) -> (w383:T13)
        n170 = call-dynamic "draw.vi"("reference"=w381, "graphics"=w369, "bounds"=w383, "ForceRedrawGrid"=w388, "error in (no error)"=w390) -> ("reference out"=w382:refnum<class "Grid.lvclass">, "error out"=w393:errorcluster)  [unwired: 13 in]
        n171 = call-dynamic "draw.vi"("reference"=w385, "graphics"=w379, "grid"=w382, "error in (no error)"=w393, "SelectedNodes"=refnum<class "AbstractNode.lvclass">[] [], "HideOverLays(False)"=TRUE) -> ("reference out"=w374:refnum<class "ClassDiagramGraph.lvclass">, "error out"=w378:errorcluster)  [unwired: 10 in, 2 out]
        n172 = call <resource>:"updateScreen.vi"("reference"=w379, "error in (no error)"=w378) -> ("error out"=w376:errorcluster)  [unwired: 17 out]
        n173 = call-dynamic "Destroy.vi"("reference"=w374, "error in (no error)"=w376) -> ("error out"=w375:errorcluster)  [unwired: 16 in, 1 out]
      }
      frame "PlaceControls" {
        n174 = Unbundle By Name(w407) -> ("CtrlRefs"=w408:refnum<vi>[], "ClassNodes"=w415:T3[])
        n175 = property on="Picture" class="Pict"() -> ("Left"=w421:i32, "Top"=w417:i32)  [unwired: 2 in, 2 out]
        n176 = Subtract(x=w419, y=25) -> (x-y=w416:i32)
        n177 = Add(x=w421, y=w420) -> (x+y=w406:i32)
        n178 = Add(x=w417, y=w416) -> (x+y=w414:i32)
        n179 = Add(x=w406, y=3) -> (x+y=w404:i32)
        n180 = for {
          tunnel: w408 -> [w442] mode=indexing
          tunnel: w415 -> [w441] mode=indexing
          tunnel: w404 -> [w438]
          tunnel: w414 -> [w435]
          shift-right: [w432] -> w410
          shift-left: w413 -> [w433]
          n181 = Unbundle By Name(w441) -> ("X"=w440:i32, "Y"=w437:i32)
          n182 = Add(x=w440, y=w438) -> (x+y=w439:i32)
          n183 = Add(x=w437, y=w435) -> (x+y=w436:i32)
          n184 = property class="Ring (strict)"(reference=w442, error in=w433, "Visible"=TRUE, "Left"=w439, "Top"=w436, "Value"=u16 0, "Disabled Items []"=i32[] []) -> (error out=w432:errorcluster)  [unwired: 1 out]
        }
        n185 = Empty Array?(array=w412) -> (empty?=w411:bool)
        n186 = Unbundle By Name(w407) -> ("ClassSelected"=w403:bool[])
        n187 = case shown="False" w411 {
          tunnel: w410 -> [w426 w430]
          tunnel: [w426 w430] -> w409
          tunnel: w408 -> [w427 _]
          tunnel: w403 -> [w425 _]
          frame False {
            n188 = Index Array(array=w427) -> ()  [unwired: 1 in, 1 out]
            n189 = Search 1D Array(1D array=w425, element=TRUE) -> (index of element=w423:i32)  [unwired: 1 in]
            n190 = case shown="0, Default" w423 {
              selector: w423 -> [w429 _]
              frame 0, Default {
                n191 = Increment(x=w429) -> (x+1=w428:i32)
                n192 = property on="Ring 1" class="Ring (strict)"("Val(Sgnl)"=w428) -> ()  [unwired: 2 in, 2 out]
              }
              frame -1 {
              }
            }
          }
          frame True {
          }
        }
      }
    }
    n193 = Equal?(x=w28, y="Exit") -> (x = y?=w31:bool)
    n194 = Select(t="Error", s=w27, f=w28) -> (s? t:f=w32:string)
  }
  "error out" <- w16
  n195 = stacked-sequence {
    tunnel: w6 -> [w444]
    tunnel: [w446] -> w4
    tunnel: [w445] -> w3
    tunnel: [w444] -> w2
    frame #0 {
      n196 = Unbundle By Name(w444) -> ("PIDs"=w450:string[], "Patterns"=w451:T15)
      n197 = local read "Design Patterns"() -> (w449:string)
      n198 = Search 1D Array(1D array=w450, element=w449) -> (index of element=w447:i32)  [unwired: 1 out]
      n199 = Index Array(array=w451, index=w447) -> (element=w448:T16)
      n200 = Unbundle By Name(w448) -> ("Nodes"=w446:T3[], "Links"=w445:T1[])
    }
  }
  "NodesOut" <- w4
  "LinksOut" <- w3
  n201 = Unbundle By Name(w2) -> ("NodeIndexies"=→"NodeIndexies":i32[])
  n202 = Unbundle By Name(w6) -> ("CtrlRefs"=w5:refnum<vi>[], "Cancelled"=→"Cancelled":bool, "Event"=w15:refnum<event-registration>)
  n203 = Unregister For Events(event registration refnum=w15) -> ()  [unwired: 1 in, 1 out]
  n204 = for {
    tunnel: w5 -> [w453] mode=indexing
    n205 = property class="Ring (strict)"(reference=w453, "Visible"=FALSE) -> ()  [unwired: 1 in, 2 out]
  }
  "GraphOut" <- "GraphIn"
